vi "Send Add View.vi"(7 "Priority":T2=enum."Normal" caption="Message Priority (Normal)", 8 "error in (no error)":errorcluster, 9 "View Details":T1, 10 "View":string, 11 "Message Enqueuer in":refnum<class "Message Enqueuer.lvclass">) -> (0 "error out":errorcluster, 3 "Message Enqueuer out":refnum<class "Message Enqueuer.lvclass">)   [LabVIEW 2023, in "GUI Views.lvlib" / "Add View Msg.lvclass"]
doc: "Sends the <b>GUI Views.lvlib:Add View Msg.lvclass</b> message.\n\nThis message will call <b>Add View.vi</b> on the <b>GUI Views.lvlib:GUI Container.lvclass</b> actor.\n\n<b>Add View.vi Description</b>\nThis method is called by the a contained GUI View to allow the GUI Container to store the GUI VIew details"
uses:
  Add View Msg.lvclass
  Add View Msg.lvclass/Add View Msg.ctl
  <vilib>/ActorFramework/Message Enqueuer/Message Enqueuer.lvclass
  C:/Program Files/National Instruments/LabVIEW 2023/vi.lib/ActorFramework/Message/Message.lvclass
  C:/Projects/Shared Libraries/Event Actors/GUI Views/GUI Container Messages/Add View Msg/Add View Msg.lvclass
  <vilib>/ActorFramework/Message Enqueuer/Message Priority.ctl
  GUI Container/typedefs/View Details.ctl
  GUI Container/GUI Container.lvclass
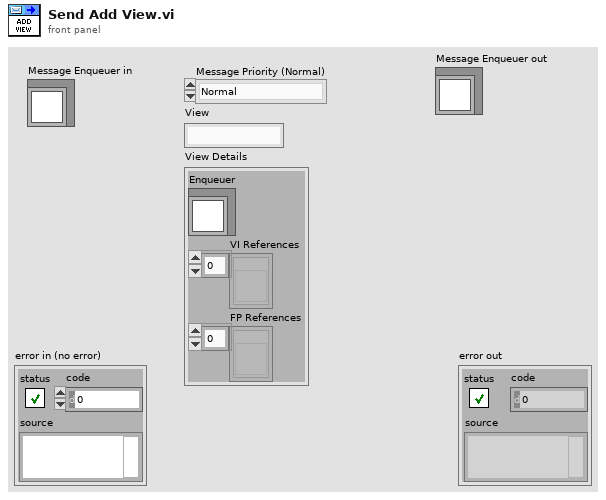
[diagram p1: front panel]
types:
  T1 = typedef "GUI Views.lvlib/GUI Container.lvclass/View Details.ctl" = cluster{"Enqueuer":refnum<class "Message Enqueuer.lvclass">, "VI References":refnum<vi>[], "FP References":refnum<vi>[]}
  T2 = typedef "Actor Framework.lvlib/Message Enqueuer.lvclass/Message Priority.ctl" = enum16{"Low", "Normal", "High"}
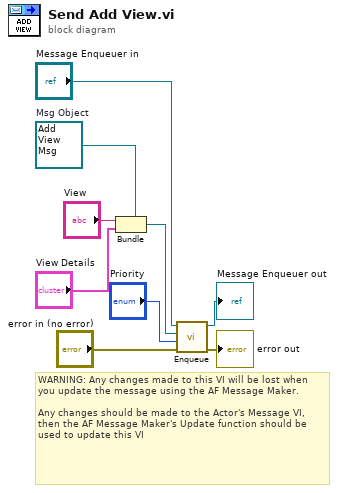
[diagram p0: block diagram]
diagram:
  w7 = refnum<class "Add View Msg.lvclass"> refnum  # Msg Object
  # "WARNING: Any changes made to this VI will be lost when you update the message using the AF Message Maker.\n\nAny changes should be made to the Actor's Message VI, then the AF Message Maker's Update function should be used to update this VI"
  n1 = Bundle(cluster=w7, "View", "View Details") -> (w2:refnum<class "Add View Msg.lvclass">)
  n2 = call <vilib>:"Enqueue.vi"("error in (no error)"="error in (no error)", "Message Priority (Normal)"="Priority", "Message"=w2, "Message Enqueuer in"="Message Enqueuer in") -> ("error out"=→"error out":errorcluster, "Message Enqueuer out"=→"Message Enqueuer out":refnum<class "Message Enqueuer.lvclass">)  [unwired: 6 in]
